vi "Untitled 1.vi"() -> ()   [LabVIEW 2018]
panel:
  out "xnor 4":bool
  out "xor 4":bool
  out "nor 4":bool
  out "nand 4":bool
  out "or 4":bool
  out "and 4":bool
  out "not 4":bool
  in  "input b 4":bool
  in  "input a 4":bool
  out "xnor 3":bool
  out "xor 3":bool
  out "nor 3":bool
  out "nand 3":bool
  out "or 3":bool
  out "and 3":bool
  out "not 3":bool
  in  "input b 3":bool
  in  "input a 3":bool
  out "xnor 2":bool
  out "xor 2":bool
  out "nor 2":bool
  out "nand 2":bool
  out "or 2":bool
  out "and 2":bool
  out "not 2":bool
  in  "input b 2":bool
  in  "input a 2":bool
  in  "stop":bool
  out "xnor":bool
  out "xor":bool
  out "nor":bool
  out "nand":bool
  out "or":bool
  out "and":bool
  out "not":bool
  in  "input b":bool
  in  "input a":bool
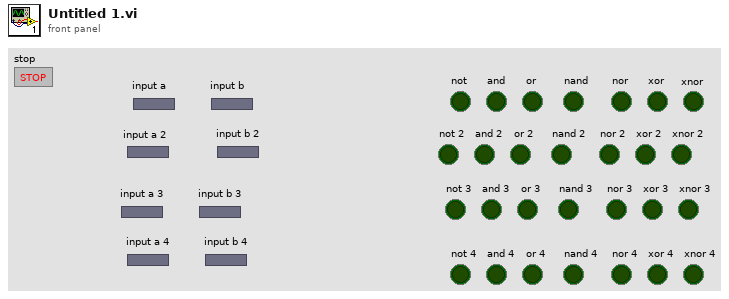
[diagram p1: front panel]
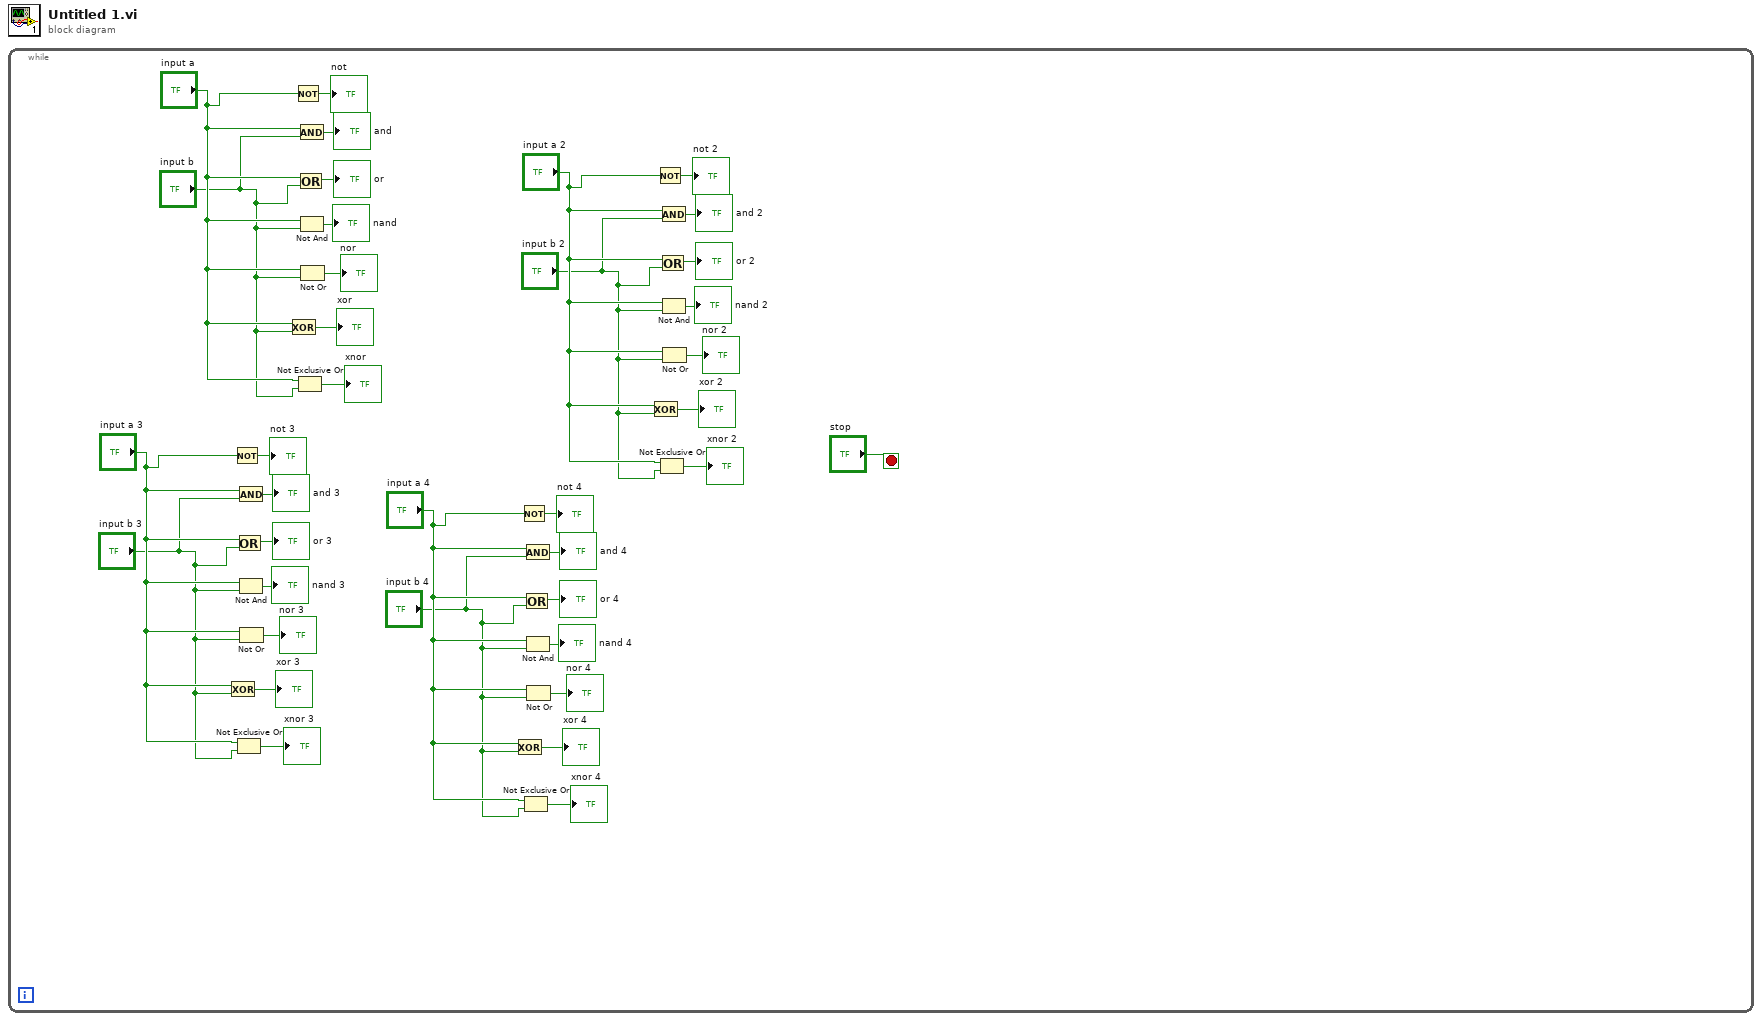
[diagram p0: block diagram]
diagram:
  n1 = while {
    stop <- "stop" stop-if-true
    n2 = Exclusive Or(1:"input b 3", 2:"input a 3") -> (0:→"xor 3":bool)
    n3 = Not(x="input a 3") -> (.not. x?=→"not 3":bool)
    n4 = Not Exclusive Or(1:"input b 3", 2:"input a 3") -> (0:→"xnor 3":bool)
    n5 = Or(x="input a 3", y="input b 3") -> (x .or. y?=→"or 3":bool)
    n6 = And(x="input a 3", y="input b 3") -> (x .and. y?=→"and 3":bool)
    n7 = Not And(1:"input b 3", 2:"input a 3") -> (0:→"nand 3":bool)
    n8 = Not Or(1:"input b 3", 2:"input a 3") -> (0:→"nor 3":bool)
    n9 = Exclusive Or(1:"input b", 2:"input a") -> (0:→"xor":bool)
    n10 = Not(x="input a") -> (.not. x?=→"not":bool)
    n11 = Not Exclusive Or(1:"input b", 2:"input a") -> (0:→"xnor":bool)
    n12 = Or(x="input a", y="input b") -> (x .or. y?=→"or":bool)
    n13 = And(x="input a", y="input b") -> (x .and. y?=→"and":bool)
    n14 = Not And(1:"input b", 2:"input a") -> (0:→"nand":bool)
    n15 = Not Or(1:"input b", 2:"input a") -> (0:→"nor":bool)
    n16 = Exclusive Or(1:"input b 4", 2:"input a 4") -> (0:→"xor 4":bool)
    n17 = Not(x="input a 4") -> (.not. x?=→"not 4":bool)
    n18 = Not Exclusive Or(1:"input b 4", 2:"input a 4") -> (0:→"xnor 4":bool)
    n19 = Or(x="input a 4", y="input b 4") -> (x .or. y?=→"or 4":bool)
    n20 = And(x="input a 4", y="input b 4") -> (x .and. y?=→"and 4":bool)
    n21 = Not And(1:"input b 4", 2:"input a 4") -> (0:→"nand 4":bool)
    n22 = Not Or(1:"input b 4", 2:"input a 4") -> (0:→"nor 4":bool)
    n23 = Exclusive Or(1:"input b 2", 2:"input a 2") -> (0:→"xor 2":bool)
    n24 = Not(x="input a 2") -> (.not. x?=→"not 2":bool)
    n25 = Not Exclusive Or(1:"input b 2", 2:"input a 2") -> (0:→"xnor 2":bool)
    n26 = Or(x="input a 2", y="input b 2") -> (x .or. y?=→"or 2":bool)
    n27 = And(x="input a 2", y="input b 2") -> (x .and. y?=→"and 2":bool)
    n28 = Not And(1:"input b 2", 2:"input a 2") -> (0:→"nand 2":bool)
    n29 = Not Or(1:"input b 2", 2:"input a 2") -> (0:→"nor 2":bool)
  }
